vi "Untitled 1.vi"() -> ()   [LabVIEW 2019]
uses:
  <vilib>/sound2/lvsound2.llb/Sound Data Format.ctl
  <vilib>/sound2/lvsound2.llb/Sound File Info (path).vi
panel:
  out "sound format 2":T1={"sample rate (S/s)"=22050.0, "number of channels"=2, "bits per sample"=16}
  out "1/x":dbl
  out "dt":dbl
  out "Waveform Graph":waveform(dbl)(graph)
  in  "Path 2":path
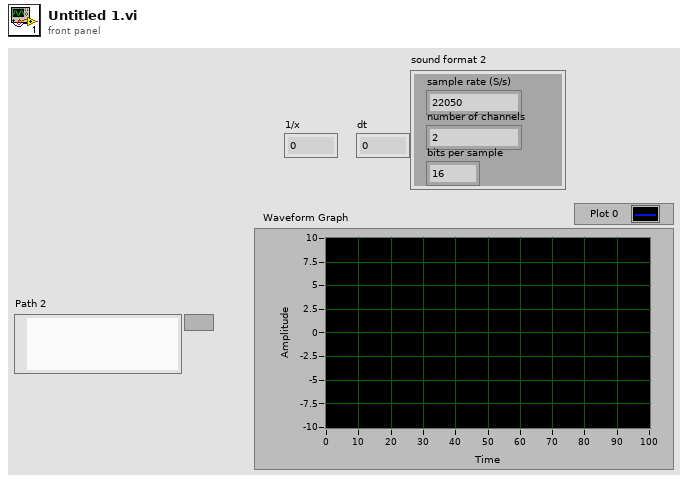
[diagram p1: front panel]
types:
  T1 = typedef "Sound Data Format.ctl" = cluster{"sample rate (S/s)":dbl, "number of channels":i32, "bits per sample":i32}
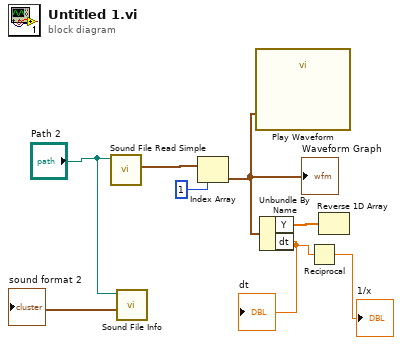
[diagram p0: block diagram]
diagram:
  n1 = call <vilib>:"Sound File Read Simple.vi"("path"="Path 2") -> ("data"=w8:waveform(dbl)[])  [unwired: 7 in, 3 out]
  n2 = call-poly <vilib>:"Sound File Info.vi"("path"="Path 2") -> ("sound format"=→"sound format 2":T1)  [unwired: 7 in, 3 out]
  n3 = Index Array(array=w8, index=1) -> (element=w6:waveform(dbl))
  "Waveform Graph" <- w6
  n4 = call "Play Waveform"("Data"=w6) -> ()  [unwired: 18 in, 1 out]
  n5 = Unbundle By Name(w6) -> ("Y"=w5:dbl[], "dt"=w4:dbl)
  "dt" <- w4
  n6 = Reciprocal(x=w4) -> (1/x=→"1/x":dbl)
  n7 = Reverse 1D Array(array=w5) -> ()  [unwired: 1 out]
